vi "DoubleQuoteIfContainsSpecialCharacter.vi"(10 "special character (.)":string=".", 11 "string in":string) -> (3 "string out":string)   [LabVIEW 2017]
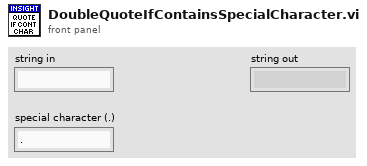
[diagram p1: front panel]
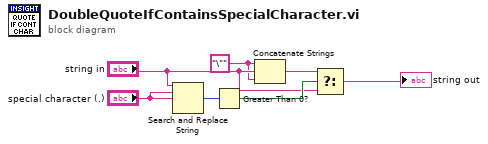
[diagram p0: block diagram]
diagram:
  w1 = "\"" ("string")
  n1 = Search and Replace String(input string="string in", search string="special character (.)", replace string="special character (.)") -> (number of replacements=w5:i32)  [unwired: 5 in, 3 out]
  n2 = Greater Than 0?(x=w5) -> (x > 0?=w6:bool)
  n3 = Concatenate Strings(w1, "string in", w1) -> (w3:string)
  n4 = Select(t=w3, s=w6, f="string in") -> (s? t:f=→"string out":string)
